vi "setTimestampFIFO.vi"(10 "TimestampFIFO":refnum<class "IReadU64FIFO.lvclass">, 11 "RTDisplacement in":refnum<class "RTDisplacement.lvclass">) -> (3 "RTDisplacement out":refnum<class "RTDisplacement.lvclass">)   [LabVIEW 2016, in "RTDisplacement.lvlib" / "RTDisplacement.lvclass"]
uses:
  RTDisplacement.lvclass
  Common_RT_FPGA/IReadU64FIFO/IReadU64FIFO.lvclass
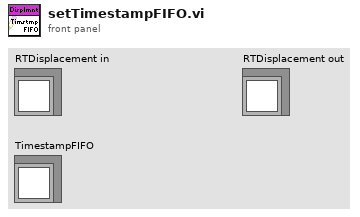
[diagram p1: front panel]
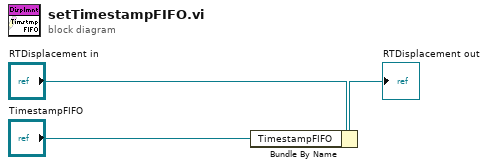
[diagram p0: block diagram]
diagram:
  n1 = Bundle By Name(cluster="RTDisplacement in", "TimestampFIFO"="TimestampFIFO") -> (→"RTDisplacement out":refnum<class "RTDisplacement.lvclass">)
